vi "UnCompress Image (HOST) (SubVI).vi"(0 "Data Array":u8[](array[numeric]), 2 "Bit Depth Array":u8[](array[numeric]), 4 "Min. Array":u8[](array[numeric]), 6 "N Bits/Pixel":u8=8, 8 "Block Size":i32, 10 "Image Width":i32, 12 "Image Height":i32) -> (14 "Image Array Out":u8[][](array[numeric]))   [LabVIEW 2014]
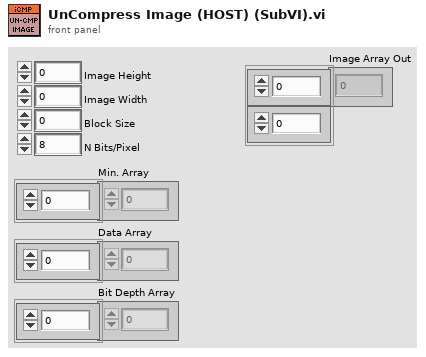
[diagram p1: front panel]
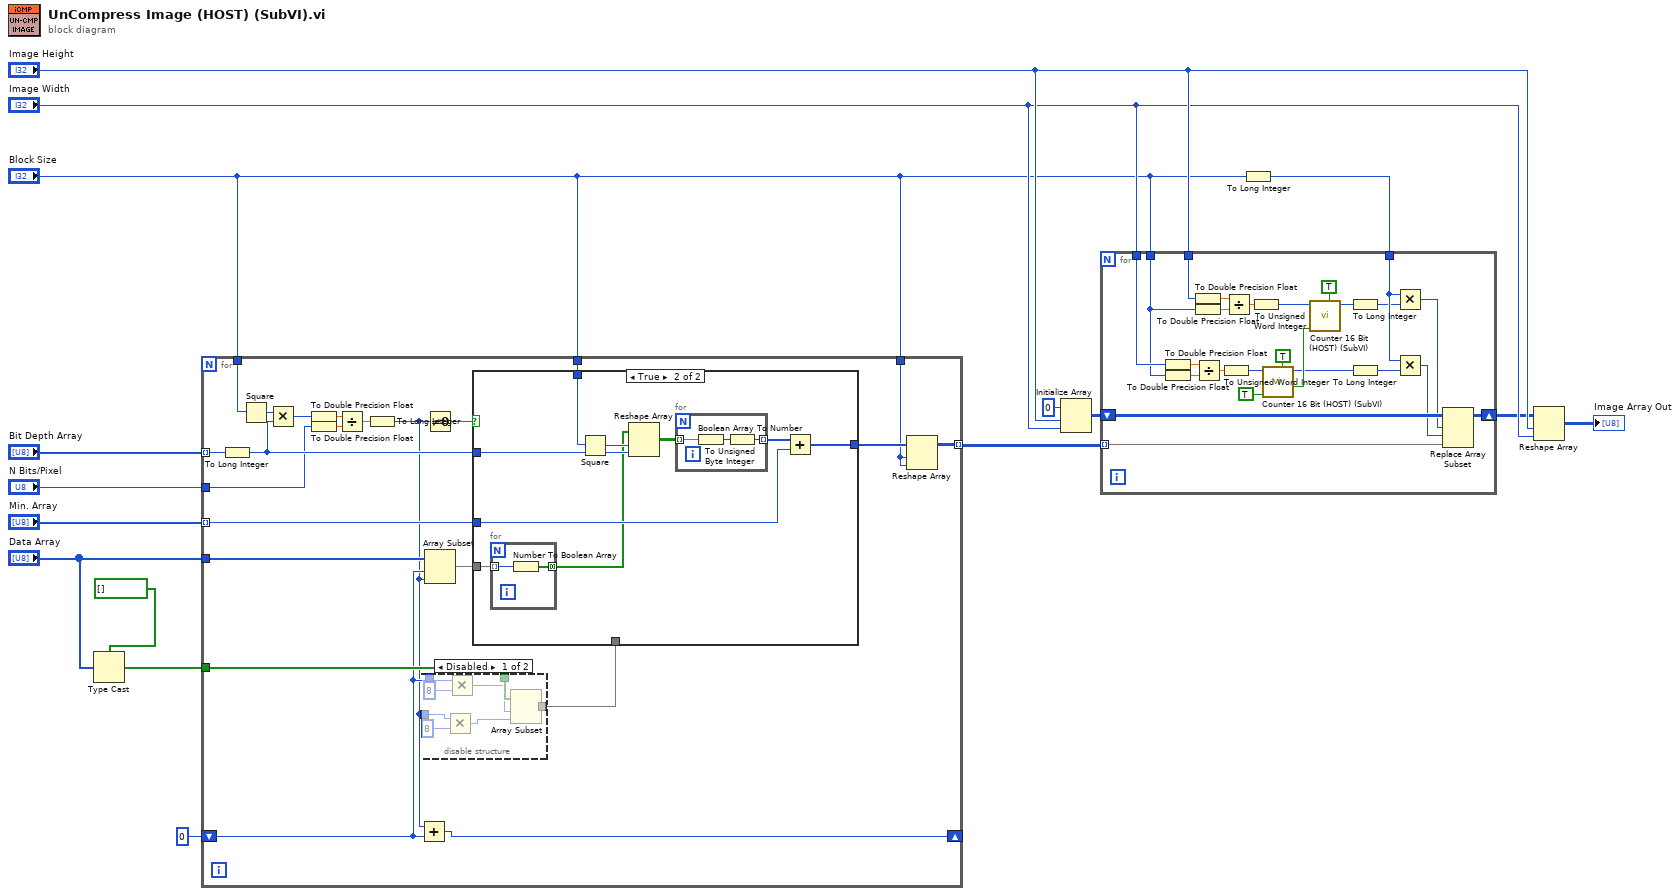
[diagram p0: block diagram]
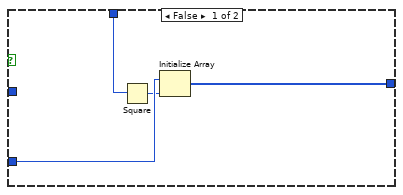
[diagram p3: hidden frame]
diagram:
  n1 = Type Cast(type=bool[] [] ("Boolean array"), x="Data Array") -> (*(type *) &x=w1:bool[])
  n2 = for {
    tunnel: "Min. Array" -> [w34] mode=indexing
    tunnel: "Bit Depth Array" -> [w33] mode=indexing
    tunnel: "Data Array" -> [w38]
    shift-right: [w37] -> _
    shift-left: 0 ("y") -> [w18]
    tunnel: [w31] -> w7 mode=indexing
    tunnel: "Block Size" -> [w26]
    tunnel: "Block Size" -> [w27]
    tunnel: "Block Size" -> [w23]
    tunnel: "N Bits/Pixel" -> [w22]
    tunnel: w1 -> [w20]
    n3 = To Long Integer(number=w33) -> (32bit integer=w24:i32)
    n4 = Square(x=w26) -> (x^2=w25:i32)
    n5 = Multiply(x=w25, y=w24) -> (x*y=w30:i32)
    n6 = To Double Precision Float(number=w30) -> (double precision float=w28:dbl)
    n7 = To Double Precision Float(number=w22) -> (double precision float=w21:dbl)
    n8 = Divide(x=w28, y=w21) -> (x/y=w29:dbl)
    n9 = To Long Integer(number=w29) -> (32bit integer=w17:i32)
    n10 = Add(x=w17, y=w18) -> (x+y=w37:i32)
    n11 = disable-structure shown="Disabled" {
      disable-tunnel: w20 -> [w46 _]
      disable-tunnel: [w45 _] -> w19
      disable-tunnel: w18 -> [w44 _]
      disable-tunnel: w17 -> [w40 _]
      frame Disabled {
        n12 = Multiply(x=w40, y=8) -> (x*y=w39:i32)
        n13 = Multiply(x=w44, y=8) -> (x*y=w42:i32)
        n14 = Array Subset(array=w46, index=w42, length=w39) -> (w45:bool[])
      }
      frame Enabled {
      }
    }
    n15 = Not Equal To 0?(x=w17) -> (x != 0?=w32:bool)
    n16 = Array Subset(array=w38, index=w18, length=w17) -> (w36:u8[])
    n17 = case shown="True" w32 {
      tunnel: w36 -> [_ w52]
      tunnel: [w49 w58] -> w35
      tunnel: w34 -> [w50 w57]
      tunnel: w24 -> [_ w55]
      tunnel: w23 -> [w48 w53]
      tunnel: w19 -> [_ _]
      frame False {
        n18 = Square(x=w48) -> (x^2=w47:i32)
        n19 = Initialize Array(w50, w47) -> (w49:u8[])
      }
      frame True {
        n20 = for {
          tunnel: w52 -> [w61] mode=indexing
          tunnel: [w60] -> w51 mode=concatenating
          n21 = Number To Boolean Array(number=w61) -> (Boolean array=w60:bool[])
        }
        n22 = Square(x=w53) -> (x^2=w54:i32)
        n23 = Reshape Array(w51, w54, w55) -> (w56:bool[][])
        n24 = for {
          tunnel: w56 -> [w64] mode=indexing
          tunnel: [w62] -> w59 mode=indexing
          n25 = Boolean Array To Number(Boolean array=w64) -> (number=w63:u32)
          n26 = To Unsigned Byte Integer(number=w63) -> (unsigned 8bit integer=w62:u8)
        }
        n27 = Add(x=w59, y=w57) -> (x+y=w58:u8[])
      }
    }
    n28 = Reshape Array(w35, w27, w27) -> (w31:u8[][])
  }
  n29 = Initialize Array(u8 0 ("element"), "Image Height", "Image Width") -> (w9:u8[][])
  n30 = To Long Integer(number="Block Size") -> (32bit integer=w14:i32)
  n31 = for {
    tunnel: w7 -> [w83] mode=indexing
    shift-right: [w88] -> w10
    shift-left: w9 -> [w89]
    tunnel: w14 -> [w80]
    tunnel: "Image Width" -> [w74]
    tunnel: "Image Height" -> [w69]
    tunnel: "Block Size" -> [w68]
    n32 = To Double Precision Float(number=w74) -> (double precision float=w75:dbl)
    n33 = To Double Precision Float(number=w68) -> (double precision float=w76:dbl)
    n34 = To Double Precision Float(number=w69) -> (double precision float=w72:dbl)
    n35 = To Double Precision Float(number=w68) -> (double precision float=w71:dbl)
    n36 = Divide(x=w75, y=w76) -> (x/y=w77:dbl)
    n37 = To Unsigned Word Integer(number=w77) -> (unsigned 16bit integer=w73:u16)
    n38 = Divide(x=w72, y=w71) -> (x/y=w70:dbl)
    n39 = To Unsigned Word Integer(number=w70) -> (unsigned 16bit integer=w67:u16)
    n40 = call "Counter 16 Bit (HOST) (SubVI).vi"("Auto RESET"=TRUE, "Enable"=TRUE, "Max. Count"=w73) -> ("Count End?"=w87:bool, "Count"=w85:u16)  [unwired: 6 in, 1 out]
    n41 = call "Counter 16 Bit (HOST) (SubVI).vi"("Auto RESET"=TRUE, "Enable"=w87, "Max. Count"=w67) -> ("Count"=w84:u16)  [unwired: 6 in, 2 out]
    n42 = To Long Integer(number=w84) -> (32bit integer=w79:i32)
    n43 = To Long Integer(number=w85) -> (32bit integer=w78:i32)
    n44 = Multiply(x=w80, y=w79) -> (x*y=w82:i32)
    n45 = Multiply(x=w80, y=w78) -> (x*y=w81:i32)
    n46 = Replace Array Subset(array=w89, new element=w83, index (row)=w82, index (col)=w81) -> (w88:u8[][])
  }
  n47 = Reshape Array(w10, "Image Height", "Image Width") -> (→"Image Array Out":u8[][])
